vi "6_1.vi"() -> ()   [LabVIEW 2023, in "2025.lvlib"]
uses:
  2025.lvlib
  <userlib>/_OpenG.lib/string/string.llb/Trim Whitespace (String)__ogtk.vi
  <userlib>/_OpenG.lib/string/string.llb/openg_string.lvlib
panel:
  out "array w/ subset deleted":string[][](array[string])
  out "Numeric 2":i32
  out "Numeric":i32
  out "sum 2":u64
  out "Array 3":u64[](array[numeric])
  out "output 2":string
  out "number":u64
  out "error out":errorcluster
  out "output 1":string
  out "transposed array":string[][](array[string])
  out "Character Array":string[][](array[string])
  out "Array 2":string[](array[string])
  out "Array of Strings 2":string[][](array[string])
  out "sum":u64
  out "Array":u64[](array[numeric])
  out "Array of Strings":string[](array[string])
  in  "Boolean":bool
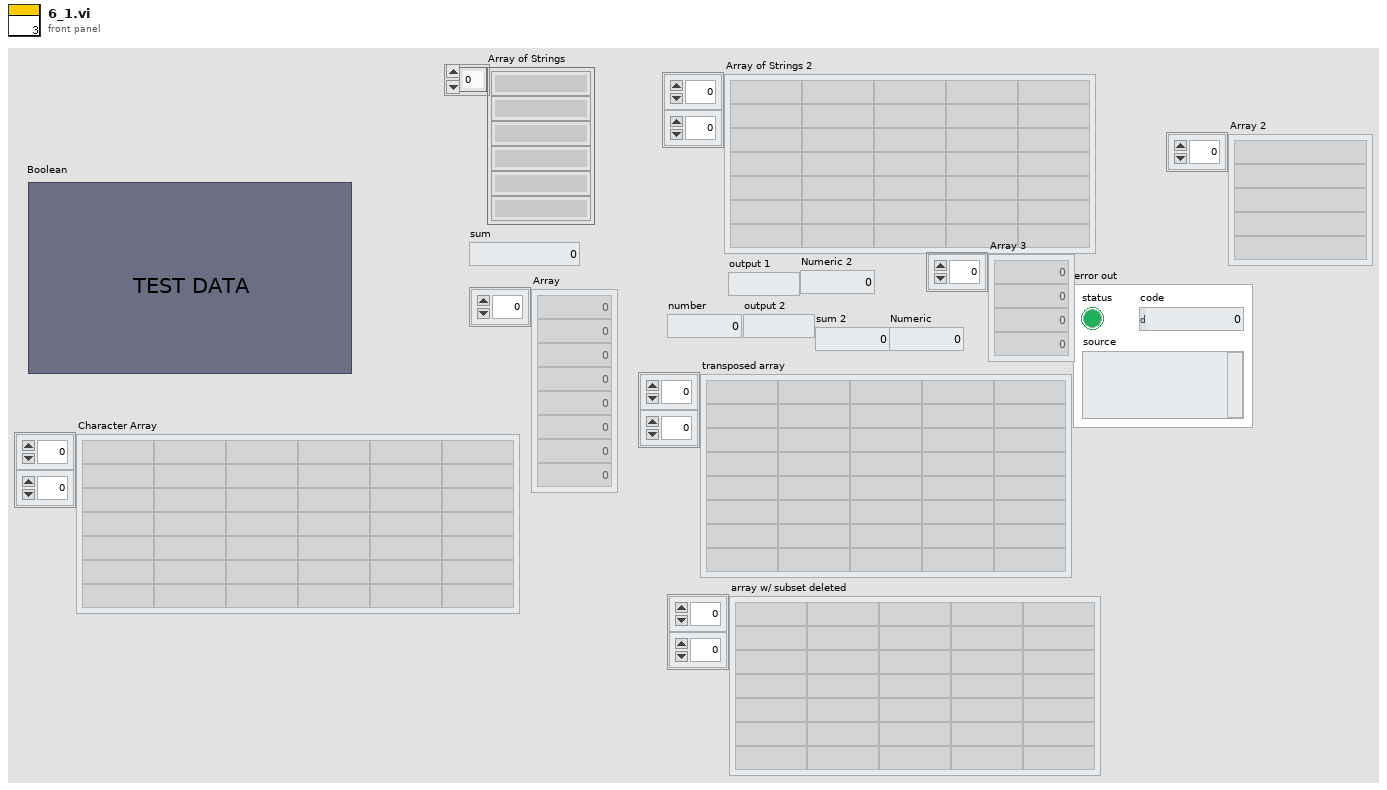
[diagram p1: front panel]
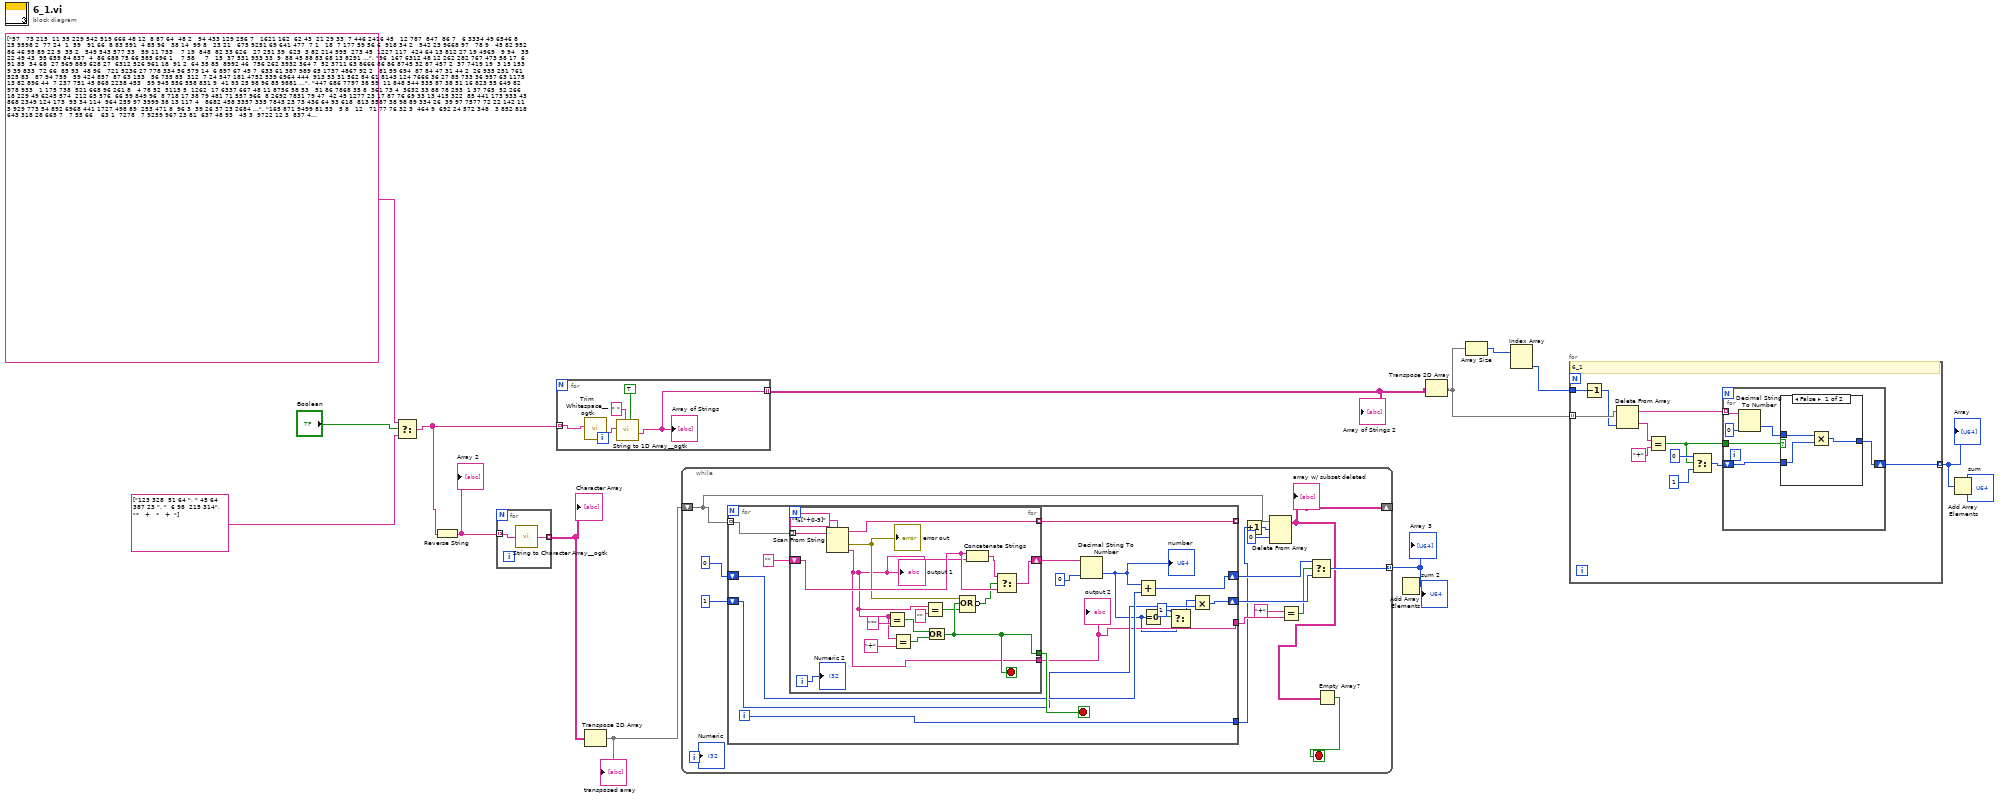
[diagram p0: block diagram]
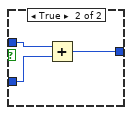
[diagram p2: hidden frame]
diagram:
  n1 = Select(t=string[] ["57   73 215  11 35 229 542 519 666 48 12  8 87 64  48 2   94 433 129 256 7   1621 162  62 43  21 29 33  7 446 2416 45   12 787  847  86 7   6 3334 49 6546 8  25 9598 2  77 24  1  59   91 66  8 83 591  4 85 96   38 14  99 8   23 21   675 9251 69 641 477  7 1   18  7 177 59 56 6  918 34 2   942 23 9668 97   78 9   45 82 952  86 46 95 89 22 9  35 2   549 543 577 33   59 11 733    7 19  848  82 33 626   27 251 39  623  3 82 214 595  273 45  1227 117  424 64 13 812 27 19 4969   9 94   35 22 49 43  95 659 84 837  4  86 688 75 66 585 696 1    7 58     7   15  37 531 933 33  9  88 45 88 83 68 13 8291 326 14  69   4 5   613 874 245  76 799 183 42  257 391  2  56 95 43 15    5  4 24  966  3 412 5  264  52 15 3  434 242  191 82    9   1 515 846   922 76   15 6281   1 59 73  9    62 18  74 82 72 6  844  8  18  898   7   33 847 4977 38 24 23 39  7 5561    9 9  93   9 417 971 77  26 89  7 5641 1  211 7  459 47 9   6    32  8 975 58 29 143 372 955   1 968  9 452  5 5  71  42 29 172 54 77  76   469  1 4352 956 3669 926 8381  1  916   2 44 536 161 3    78  4 4546 8   53 866   74  86  4 2  478 32 8   917  533 75 869 9   33  93 583 67 434  66 926  12 737 981 4    8 536  2674 3    6332 1515   4 24  1 982 717 41 26 64 5  53 432 662  815 486 147 6   4 87 84 2712 4   793  89 2164 539 675   59 96 6888  1 373   1  16 721 97  54 16 759 66 8  5    948 17  6  8  45 923 4664 36  4 62 624 73 494 73 171 312 98  3 288 63    9 7351 69    44  4   8   3  2 414 942  62  1  3 528 83 779 158 1  781 27  946 879  21   8 895  24  327 49 39  33 2361 58 15 325 89 82 76   99 845 7981 241   6 3377 12 72 543 837 5647 566 298 6293    3 8974 456 957 2    871 2197 993 13   66 8853 6  1  246 5    9   97 56 552  233   8 955 86 52   3 9   4  5  57 62 239 3  57 339 7  754 43 55 8663 242  68 33 79 4617  3 9  782 37 119 1  24  865 319 5   16 335 824   5 591 14   1   1 483 39   7 478 99 3815 97  77 176  5 2499 4935  52 841  71 181 96  4 76 59 888 61 3363 21 565  7 7   38  591 79  4    1 16   37  27 58 79  77 1   578  75 54 6   55  7 142  41   19 97 753 918 786 94  2     4  3 882   6 4352 92 975  7 691  268 74 819   54 6   2  54   94 6341 35  738  73 89 6  53 19  6791 63 339 12 78 2   9 35  697  56 132 84 95 8611 37 16 144 8  66 61 512 2  919  613   1  9 95 68 489 225 576 222 9  769 3374 95 35 53 25 222 638 4    1 84 1  56   8 57 182 443 797 136 9    9   8 53   53 3  3721 79 15 583   16 335 23 7158 564  4  9 65 72 3719 891 683 3769  83 233  771 51 811 65 4  7567 5842  93  83 23 32 935 77   6976 26  52 53 549 8936 76 1  6   5  6   872  7 83 3376 512 61 59 354  5367  4 9434 56 67    5 9  32    3 5846  7 5  9    98 535 12  37   1 7846 62 41 73 63 894 3   9 635 3724  96  16 11 51 69 495 15 97 54 536    5 987 82 353  6 939 72 389  53 52 11   4 344 3   782 5    228 657 328 543  516  4 348 5629   13 447 666   8 95 832 291 411  74  19 39 483  9 88 11   46 37 56  74 25  6683 1157 616 73 9  86  71 71   59 7    4  37 14 348 559 76 987  78 55 5  14 443 7682 1   1721 516 91   836 464 634 44 7428 64  471 218 646   9  2 57 9    183 71 46  17 917 12 13   235  5 488 4566 953 191 42  1 481 63 9  344 28  253 116 19  74 12 57  8 1697 15 9414 54   25 213 33 515 95 11  6183 23 814  396 4  66 663  7 29 266  81 335 84  5 5284 7  23 63 454 778 3926 696 4    74 84 2584  95 763 528 565 7  962  2  12 64 71   9 5  13 272 374 73 17 58 985 2   14 47 56 5    27  69   23 48 24  229 75 8429 7546 98   6 86 9974 151 6918 77 798 12 862 565 7157  92 848 45  79 48 69 741 96  45   818 35 96 9246 542 9486    9 152 9  41 881  38 292  77 6   3  9  4  5  81 94   62 327 97  35  3824 426 3   7    88 537 543 921   6 95  471 113   36 3  31 761   7 7934 8787 317  2 7996 35 38 649 24  29 6717 53 25   892 24 846 74  4 661 54 2238 6993 61 93 16   6 962 78 67 4   958  45 395 393 2   95  338 38   865  7 7318", "96  167 6312 48 12 262 282 767 473 58 17  6 91 85  34 68  27 569 889 628 27  6312 526 961 18  91 2  64 35 85  8992 46  756 262 3932 364 7  52 3711 63 8666 86 86 8745 32 87 457 2  37 7419 19  3 15 153  9 39 833  72 66  85 93  48 96   721 5236 27 778 334 56 579 14  6 897 67 45 7  633 61 387 989 65 1737 4867 92 2   81 59 694  87 84 47 31 44 2  26 935 251 761 525 83   87 94 759   59 424 857  87 63 153   56 735 85  312  7 24 547 181 4752 539 6964 444  913 53 31 562 84 61 8143 124 7666 36 27 85 733 36 957 63 1175 13 82 896 44  7 237 751 45 868 2238 453   59 945 556 558 831 9  41 93 25 98 96 85 9881 836 761 55  79 85 3122 327 2117 83 386 292 88  457 235 72  99 94 99 45  266 44 85   55 68 72  8  587 848 7  8   16 811 2697 362  48  66 413 7369  584 21  796 7819  41 57 31  93   39 52  26 57 82 89 657  1  217 243  99  817 648 5217 41 63 14 61 38 6165 4754 7  98 783 626 153 24 478 39  6 6187 56 361 47 468 49 37  38  495  1 873 26 65  36 641 479  51 472 96 192  9 1  39  18 24 211 49 72  31  3878  8 3547 33  5588 964 1169  6 7481  28 75 682 321 4    59 28 1821 87  92 154   74  91  9 59 92  27 93  419  292 31 553 99  76  62 733 54 765  23 669  44 478 84  8   56 679  7426 98   9569 7284 678 55  6 785 114 5  66 34 3  74 527 118  151 146 547 81 34 23 93 9478 1   965 824 9313 768 59   974 38 3868 82 571   9  55 249 664 74 28  29 37 23 364  888 71  2 76 756 648 8179 59  9 41 781 44 838 33 132 492 37 23 577 9197  2 3447 3261 626  2 849 759 51 993 254  77 37  8 716 79 198 419 42 242 27 1356 2515 15   4 162  18  675 47 96  46 581  43 91 393 25 93 87   26 483 4614 337  45   99  7 84  63 888 7676 236  95 5241    6 5181 142 914 5952 634 4579 685 57 7715 3659 4  8  662 97   1 1942 47 6876 249 347 491 95 79   7 8   18 3  62 52 537 51 65 532 17  81 97 81 1324 611  24 32 49 7996  3 92 516 19 472 8  31 6255  15 4   18 773 285 794 317 21   9   5 252 51   5 41  53 2396 53 489 764 88 3767  919  85 518 842 633 92  3 19 58 246 97 9315 33 523  7 611 89   31 755 77  65 6659 38 946 17 68 513 23  478  62 35 843 54 85 464  87 3387 25  99 298 497 113 126  44 55 71   27 7164 59 525  2 416  327 24 285 7122 62  2  636  53 4842 12  365  28 43 6  53 32  489  24 828 77 22 12  9 812 793  31 221 81 79  832 97 94 834 7  52 96 976 15 9616 899  77 49 14 35 839 921 398 926 5  474  615 53 77 94  8  83 736 43   8 43 1  63  63 19 382 882 316 222 41   34 36 74   95 9  2138 15 36 818  281 536 95 7653 631 22 97 39 11 4482 784 978 6338  47 2737 235 31 495 88 4   814 5282 355 414 41 73 942 158  7598 32  19 55 323 398  92 95 98  33 59  619  7 56 6231 926 68 28 284  6973  6 5937 11 194  72 3  652 319  577 72 25 216 689 658 27 828 476 9578 67 94 65 35 442 12 72 843 5432  61  16 94 98 46 382 56 34 31 754  126 928 42 522  9 439 77 849 826 81 22   4 422 76  478 629  563 315 856  41 4157  1 86  1146  381  33 669  78 91 117 324 587 753 495 57 591  5 66 449  66 82 94  29 592 4254 7359 413 67 6  72  25 587  61 5    3 358 36 177 478 34 318 374 12 7  21 288 7239 459 5779 678 967  995  12 994 44 3931 69  933 635 439  88 88 32 5    986 53 171 45 454 58 8849 199  9 942 1211 724 793 21 76 932 67 75 291 75  835 292 92  59 55 31 84 1749 72 2246 74   58  99 29 225 49 882 4972 98 425  251 33 61 932  2 14 543  62 325 21 19 2335 8  47 16 324 194  786 966 63  117 64 4588 617 415 763 977 98 185 84 926 28 14  11 6  18 252 529 2  96 43 136 37  53 93 13 725  39  11  167 98 49  718 71  246 1646 45  44 77 9887 577 9281 67 894 16 514 122 2352 453 662 95 426 99 16 919 323 797  353 17 63 2163 595  644  564 758 26 73 566 333 523 143 571 5  27 53 5  85 848 285 526 545 149 9986  38 71  6167 6  784 619 527  77 39  659 1373 238 3  15 163  23 5592 6824  92  5 3299 62 71 721 469 39 1284 62 53  6314 68 51  84 56 876 23 6488 3433 55 12 85  45 353 64 96 52  567  62 811 948 46  61  94  1276 456  1  979", "447 686 7797 38 59  11 848 544 535 87 38 51 16 823 55 649 82 978 933   1 175 738  521 668 96 261 8   4 78 52  5115 5  1262  17 6337 667 48 11 8756 58 53   51 86 7868 35 8  361 73 4  3632 33 88 78 293  1 37 765  52 266 18 229 49 6245 574  212 65 576  66 59 849 96  8 718 17 38 79 481 71 557 966  8 2692 7831 79 47  42 45 1277 23 17 87 76 69 33 13 415 322  85 441 173 933 43 868 2349 124 173  93 34 114  964 259 97 3999 38 13 117 4   8682 458 3357 335 7843 23 73 436 64 93 618  813 5587 38 98 89 334 26  39 97 7577 72 22 142 11  5 929 773 54 892 6968 441 1727 498 89  253 471 8  96 3  39 26 37 23 2684 779 333 13 667 83 3443 247 7239  1 942  73  8  398 39  72 267 72 14 629 656 92 52   94 37 7   4   61 851 3  55  67 852 8193 3439 37  38  53 3651 2548 22 5211 4494 226 96 549 6396  4 2   14 51 36 59 229  33 423 236 116 7857 288 473  75 71 49 26 42 13   3883 99 71 278 689 29  98 712 83  7  766 59 949 72 566 59 888 183 397  2 692 1   2  68 188 551 794 29  97 791 61 69 941 79 15  41 49 997 894 6199 52 4449 9   3257 142 1448 29 9852 971 34 866 684 721 854 63  679 22  22 712 3935  35 37 53 86  62 785 116 9146 64 926 974 31  73 845 36 4585 55  26 742 332 46  5  782 6599 1591 2648   11 413  443 75 62 686 614 2  73 67 4  28 227 883  132  18 166 68 57 65 16 87   64  373 895 1781 523 95  4957 66 6562 23 953  67 682 541 547 64 89  16 1  47 358 2155 51 42 99 483 579 3433 42  1 27 385 45 561 83  94 624 49 37 235 3411 35 9558 6167 447 16 591 221 85 445 387 251 52 64 866  6 623  29 33 12  59 4563 4941 525 37 4873 236 593 83 633 32 547  13 64 468 34 96 51  298 228 3375 316  38   35  2 72  78 363 9946 613  33 2983 9714 5791 66  447 4778  84 3384 81  29 5613 224  48 65 17  169 12 1291 19 3643  89 143 154 19 35   2 995 96 9  44 7  696 39 18 315 94  98 47 83  354 1636 73 33  4 36   73 14   7 16 537 33 81 7379  55 286 28 282 98  352 997 776 82 884 882 35 829 47  83 7133 62 969 543 22 5772  379 616 28  696 464 89  7 72 88 697 1  9869 68 213 91 196 622  24 166 45  38 7614 27 363 91 67 989 383 121 248 48 288 92 58 626 322 1196 32  32 971 524 956 751  65 18 54   11  442  2 21   2 994 1381  4 469 8368 692 48 954 469 5349 191   2  51  7 56 99 987 56   87 47  66 53 49  9 141 584 169 947 95 85  563 51 74 297 88 34 26   6 28 7254 847  41 56 84 56 424 314 97  323 43 326   73 95 17 69  8  54  76 941  4 54 84 23  61 49 996 917 97  857 8743 49 21 5884 45 84 3937  7 94 581 5435 246  4 4291 657 95 97  7 9   118 147 584 8217 718 5333  22 21 811 69 47  634 7366 676 888 69 14 939 541  6454  4 941 29 614 68   37 32 859 59 265  53 38 54 6997 939 33 56 794  881  44 4162 26 725 258 47 694 368  753 28 93 423 212 42  73 782 372 3676 17 62 79 64 834 76 49  49 523  227 835 84 53 65 447 42 3  84 78  6777 137 57   7  6 386 72 818 959 56 15  61 532 213 369 1133 475 824   5   5 8751 91 78  5171  872  81 4277 91 2  963 676  72 426 632 36 381  6 44 9124  3 88 23 414 556 5136 83   543 72 2  61  82 9261 54 985  4 512 25 73    5 1    1 579 47 49 45 811  976 975 2823 363 7985 458  64 571 81 2663 942  52 56   76 668 25 85 973  566 41 467 93 834 83 5426 681 85 174  316 573 93  49 12 532 55 99 865 542 281 29  866 85 29 81 12 3665 77 1994 659  86  35 26 57  54 767 3531 27 44  7773 32 68 914 57 2  127 127 843 55 48 9358 83 47 95 865 327  266 515 73 2296 99 4218 319 26  286 69  34 652 71 719 32 78 867 99 3  967 147 1  65 39 928 588 36 23  3 773  868 49 1981 62 36  436 16   68 2413 37 623 18  286 263 9775 1   59 62 298 278   51 297 228  8 738 88 97 844 544 8699 5   35  2 8257 359  123 6839  95 15 21 368 335 587 353 461 65 46 24 65 24 619 137 653 858 134  877  76 735 3314 3  148  23 87   45 756 432 2451 672 1  35 173  97 2575  361  24  4 2913 67 94  61 974 29  685 17 961 1214 61 29  26 83 378 98 184  8211 9  11 462 74 573 86 77 178 564 928  42 197 486 536 95  3348 171 49  459", "165 871 9499 81 53   5 8   12   71 77 76 32 3  464 9  692 24 572 348   3 852 818  643 318 28 665 7   7 55 66    63 1  7278   7 9259 967 23 81  637 48 93   45 3  9722 12 3  837 43 2  1494 57 58 25 177 97 54 2917 4  475 41 564 95 4118 715    9 13 618  45 44 146 43 55 7   18 66 48 7   6  754  73  1 9852 9934 84 385 34 89 5512 4  23 34 86 58 86  7 117 284  45   5 876 721 45 48  2444 881 25  635 69 34  6146 96  95 9592 26 55 384 5   6749 695 3749 714 8851 49  7 232 33  2 78   214 3388 71 15 33 763 66   6 99 4948 31  7 958 99  2 29  497 84 199 9575 894 2924 795 17  532 548 85 7  7  12 24 63 4  6626 71  725 48 282 99 8363 526 9521  4 64    9  6 3362 74  21 643 1  74 387 697 58 761   8 76 8   17   5 323 6  46   3 757 1245 9261 31 716   9 2737 2546 6  6697 9661 682 36 454 9846  8 3  681 67 27 29 2139 38 517 939 735 1532 374 599  17 31 31 94 92 86   6785 86  9 836 853 68   5 814 12 49  541 32 11  58 43  38 544 788 738 29 8   2   3   6 245 5   754 77  72 184 38 62 771 84 43  16 16 419 553 4382 65  732 7     91 653 63   66 5328 178 37 557 7   868 399 67   86 166 25 744 8795 585 62 32 95   4 341 376 3583 96 628 994 639 97  61 84 3816 47  91 395 784 53  84 886 9945 225  4277   27 5    365 5  81 528 69  3  85 77 24 22 884 2321 449   2 188 38 56 38 29 8    424 95  329 852  152 92  5857 52  653 88  53 532 357 237 813  8 22  31 8  91 341 9294 24 67 49 819 816   96  2 69 45 3   85 445 9   95 947 49 99   7 6329 11  795 9143 613 12 767 787 51 22  388 258 76 85 122  3 966   6 55 37  58 6764 8243 353 51 4153 481 499 28 398 6  82   14  4 46  99 24 32 3192   5 83   86  796   71  5 65  54  13 9683  36  48 8159 7158 53   21  235 1899  85  918 71  78 1617 982  16 33 5   968 35 7641 59 9415  85 686 9   29  8 257 199 66 34 88 4  726 49 74 115 63  41 14 83  988 6184 97 61  1 6    42 93   5 4    3 28 3  1798  46 691 27 6   87  832 711 434 12 354 815 53 676 21  8  7454 69 199 321 75  263   23 878 15  816 999 6  18 54 84 697 5  66   59 535 67 782 431  28 674 28 148 5267 28 816 33 54 686 497 819 667 34 345 9  71 336 695 1984 54  74 13  291 151 258 912 89 54  481   58  9 4   23 611 3335  8  27 1692 412 11 651 385  486 793   9 955  2 43 26 529 75   47 81  52 41 11 19 962 75  176 758 9  19    5 33 77 33  86 97 53   6 37 2491 636 852 73  9 19 867  75 79   49 53 485   14 47 89 6   9  82  56 621 21  6 65 68 767 43 76  728 25  41  2753 86 54 3553 6  85 7644  2 15 351 7374 82   3 5364 566 11 59  4 3     4 526 485 8554 494 9664   8 33 49  79 67   32 683  724 149 42 3  628 9998 2     4 523 68 325 19   96 64 714 73 754  88 83 7  4418  16 32 61 2726 28   46    7 73 364 424 25 277 245    8 28 36 113 493 66  2  916 863 6118  6 35 19 87 54  36 73  85 37   852 925 41  5 31 325 8  1  87 2   2323 898 16   7 35 656 18 688 319 13 28 469 825 334   2 9842 965 916   5   7 4724 31 18  193  8873  81 7662 33 3  217 372   4 986 951 1  41  86 36 9548  1 56 99 141 336 4757 35   175 71 72 45 851 8436 64 239 87 694 46 3     9 3    6 895 51 96 4   88    1 673 687  185 5277 587   9 6   23   56 458   1 23    4 827 63  2 7774 144 38 254 14 289 47 1542 497 38 19   948 511 7   66 17  88 5  46 498 168 658 17  169 99 56 1  55   56 79  651 1666 91   1 64 5   57 737 452  21 1   6919 21 54 931 85 3   14 738 354 45 79 2333 12 62 17  81 347  381  42 24 6465 28 2524 375 9   263 6   78 26  44 454 5  43 817 85 3  28  129 9  49 83  73 382 27 76  4 1321 891 43 8578 35 363 4   38    3  172  4 685 98   49 6   4594 3   34 72 878 435   12 967 51   1 984 93 1  8   421 7776 2    2  4  386  52  784 4968   9 75 6  569 611 722 936 345 82 55 15 22 13 986 179 633 837 443   72   5 416 1249 5  146   1 2   196 835 596 8915 992 99  4  49 587    1    3   4 73   33 84 23  82 938 97   67  9 489 1725 6  86  97 92 467 44 88      7 6  88 955 73  85 2  32 389 548 987  74  53 375 189 46  2373   5 99  818", "+   *   +    *  *  +   *   *   +   +  *  *  *  +   *  +   +  *   +   +   *   +    +   +   +  *   *  *  *  *   +    *  +    +   +    *   *  *  +    +  +    *  *  +    *  +  *   *  *  +    +  *  *  *   *  *  +    *  +   +  *   +  +    +   +    +  +   *   *  +   *  *  +   *  +  *  *   *  +   +   +  +    +    *  +   *  +  +    *  *  +  *  *  +  *  +   *   *   *   +   +   *  *   +    +   *   *   +  *   +    *   *  +    +  +  *   +   +    +   +    +   +    *  *  +   *  *  +    *   +    *  *  +  +   *  *   *  +    *  +  +   *  *  *   *   +  +   +    *   +    *   *   *   *   +  *  *  +  *  +  *  +    *   +   +  *   *  +    +   +    +  +   *   *  +    +   *  *   *  *  *   +   *  *   +   *  +   +  +   +   *  *  *   +   +    +    *  *   +   +    +    *  +    +    *   +  *   +    *  *  *   *  +  *  +    *  *   *   *   +    +   +    *  *  +  *  *  +    +    +  *  *   +   *   *  *   *  *  +    *  *   *  +   *  *   *   +   *  *   *  +  +   *   *   +   *   *  *   *  +  *   *  *  +   +  +   +   +    *  +    +   +    +   +    *  +    +   *  +   +   +   *   +  +    *   *  *   +    +   +  *  *   +  *   *   +    +  +   *   *   +  *   +  +    *  *   *   *   +   *  *   +    +    +    +    +    *   *  *  +   +   *  *  *  +  *  +   +    *   *   *   +  +  *  +  +    +   +   *   +    +   *   +    +  +    *  +   +   +   +   *   *  +  *   *  +  *   +    *  +  *  +   *   +    *  *  +  *   +  *   +  +   *   +  *  *   +    +  +    +    *   +  +   +   *  *   *   *   *  +  *   *  *   *   *  +   *  +    +    *   +  +    *   *   +  *   +  +    *  *  *   +  *  *  +    +   +    *   *   +    *  *  +   +   +    +   +   +    +    +    *   +   +    *   +    *   +  +    +    +  +  *   *   *  +    *  +    *   *   +   *  +  *   *   *  *  *  *  *   *  *  +   *  *   +  *  +    +    +  *  *  +    +  +  +   *  +   +  +  +    *   *   *  *   *   *   *   *   +  *   *   +  *   +   *  +    +  *   *   *  +    +    *   +   *   *   *  +  *  +  *   *  +    +  *   *  +   *   +   *   +  +   +    *  *   +  *  +   *   +   *   +  +   +  +  +   +   +    *  *   *   *   +   *   *   +  *   *   +    *  +   +  *   +    *  +   +    *   +  *   *   +    *   +   +   +  *  +  *   +    +  +   *  *  *  *  *   *   +   *   *  +  +    *  *  *   +  +  *  *   +  +    *   +   *  +  +  *   *   *   +   *  *   +    *  *  +  *  *   *   +   +  *  *  +  *   +  *   *   *   *   +    *  *  +    *  *  +    *  *  *   +    +   *  +    *   *  +  *  +  +    *   +   +    +   +    *   *  +   +  *  +    +    *   *   +  *  *   +    +    *  *   +  *   +    +  +  +   *  +   +   *  +  +    *   *  *  +    +    *  +    *  +   *   +  *   *   +    *  *  +   *   +   *  *   *   +    +  *  +  *  *   +  *  +   +    *   *   +  +  *  *   +  +  *  *   +    +   *  *   *  +   +  *   *   +  +  +   *   *   *   +    *   +   *   *   +    *  +   +    +    *   +    *  +  +   +   *   +   +   *  *   +  +  +    +  *  +  *   *   +    +    +   *  +  *  +   +    +  *   *  *   *  +   +   *  *   *   +  +  +  *   +    *   +    +   +    *   *   *   *  +    *   +   *   *   +   *  +  +    +   +  *   *  *   +  +    +   *  +   +    *   *   *  +  *   +  *  *   *   *   +   *   *  *  +  *  +    +  +    +    *  *   *  *   +  *   +    *  +   +    *  *  *   +  +  *   *   *   *  *  +    +  +  *  *   +   +    +   *  +    *  +    *   +   *   +   *  +   *  +   *  *  +   *  +  +   +   *  *  +  +   *   +  +  +  +    +   *  +    *  *   *   *  +    +    *  *   +  +    *   +    *  +   *  *   *   +    *   *   *  *   +  *  +   *   +    *   *  *  +    *   +    +    +   +  +  *   *   *   *   *   *  +  +  +  *  +   *   *   *   *   +    *   +   +    *  +   +   *   *   +   *   +    *   *  *  +   +   +    +    +   +  +    *  *  +   *   +  +    +  *   +    *  *   *  *  +   *  +    +    *  *  *   +  *   +  *  *   *   +   *   +   +   *   *   +    *   *  +   "], s="Boolean", f=string[] ["123 328  51 64 ", " 45 64  387 23 ", "  6 98  215 314", "*   +   *   +  "]) -> (s? t:f=w6:string[])
  n2 = Reverse String(1:w6) -> (0:w5:string[])
  "Array 2" <- w5
  n3 = for {
    tunnel: w5 -> [w17] mode=indexing
    tunnel: [w16] -> w4 mode=indexing
    n4 = call <userlib>:"String to Character Array__ogtk.vi"("Input String"=w17) -> ("Character Array"=w16:string[])
  }
  "Character Array" <- w4
  n5 = for {
    tunnel: w6 -> [w20] mode=indexing
    tunnel: [w18] -> w7 mode=indexing
    n6 = call-poly <userlib>:"Trim Whitespace__ogtk.vi"("String in"=w20) -> ("String out"=w19:string)  [unwired: 6 in]
    n7 = call <userlib>:"String to 1D Array__ogtk.vi"("ignore duplicate delimiters? (F=No)"=TRUE, "delimiter (Tab)"=" ", "string"=w19) -> ("Array of Strings"=w18:string[])  [unwired: 8 in]
    "Array of Strings" <- w18
  }
  "Array of Strings 2" <- w7
  n8 = Transpose 2D Array(2D array=w4) -> (transposed array=w3:string[][])
  "transposed array" <- w3
  n9 = while {
    shift-right: [w24] -> _
    shift-left: w3 -> [w26]
    tunnel: [w30] -> w2 mode=indexing
    i -> [w27]
    stop <- w23 stop-if-true
    n10 = for {
      tunnel: w26 -> [w51] mode=indexing
      tunnel: [w53] -> _ mode=indexing
      shift-right: [w46] -> w33
      shift-left: u64 0 -> [w47]
      shift-right: [w44] -> w32
      shift-left: u64 1 -> [w45]
      tunnel: [w43] -> w35
      tunnel: [w42] -> w28
      i -> [w42]
      stop <- w52 stop-if-true
      n11 = for {
        tunnel: w51 -> [w70] mode=indexing
        tunnel: [w69] -> w53 mode=indexing
        tunnel: [w56] -> w43
        tunnel: [w59] -> w52
        shift-right: [w62] -> w49
        shift-left: "" ("output 1") -> [w61]
        i -> [w57]
        stop <- w59 stop-if-true
        n12 = Scan From String(format string="%[*+0-9]", input string=w70) -> (remaining string=w69:string, error out=w60:errorcluster, output 1=w56:string)  [unwired: 3 in, 1 out]
        "output 1" <- w56
        "error out" <- w60
        n13 = Equal?(x=w56, y="*") -> (x = y?=w66:bool)
        n14 = Equal?(x=w56, y="+") -> (x = y?=w64:bool)
        n15 = Equal?(x=w56, y="") -> (x = y?=w54:bool)
        n16 = Or(x=w66, y=w64) -> (x .or. y?=w59:bool)
        n17 = Compound Arithmetic op=OR(w60, w59, w54) -> (invert w58:bool)
        n18 = Concatenate Strings(w61, w56) -> (w63:string)
        n19 = Select(t=w63, s=w58, f=w61) -> (s? t:f=w62:string)
        "Numeric 2" <- w57
      }
      "output 2" <- w43
      n20 = Decimal String To Number(string=w49, default (0L)=u64 0) -> (number=w40:u64)  [unwired: 1 in, 1 out]
      "number" <- w40
      n21 = Add(x=w40, y=w47) -> (x+y=w46:u64)
      n22 = Equal To 0?(x=w40) -> (x = 0?=w41:bool)
      n23 = Select(t=u64 1, s=w41, f=w40) -> (s? t:f=w38:u64)
      n24 = Multiply(x=w38, y=w45) -> (x*y=w44:u64)
    }
    n25 = Increment(x=w28) -> (x+1=w25:i32)
    n26 = Delete From Array(array=w26, length=w25, index (row)=0) -> (array with subset deleted=w24:string[][])  [unwired: 1 in, 1 out]
    "array w/ subset deleted" <- w24
    n27 = Equal?(x="+" ("y"), y=w35) -> (x = y?=w31:bool)
    n28 = Select(t=w33, s=w31, f=w32) -> (s? t:f=w30:u64)
    n29 = Empty Array?(array=w24) -> (empty?=w23:bool)
    "Numeric" <- w27
  }
  "Array 3" <- w2
  n30 = Add Array Elements(numeric array=w2) -> (sum=→"sum 2":u64)
  n31 = Transpose 2D Array(2D array=w7) -> (transposed array=w10:string[][])
  n32 = Array Size(array=w10) -> (size(s)=w9:i32[])
  n33 = Index Array(array=w9) -> (element #2=w8:i32)  [unwired: 2 in, 1 out]
  n34 = for {
    tunnel: w10 -> [w81] mode=indexing
    tunnel: [w72] -> w12 mode=indexing
    tunnel: w8 -> [w71]
    # "6_1"
    n35 = Decrement(x=w71) -> (x-1=w80:i32)
    n36 = Delete From Array(array=w81, index=w80) -> (deleted portion=w78:string, array with subset deleted=w79:string[])  [unwired: 1 in]
    n37 = Equal?(x=w78, y="+") -> (x = y?=w74:bool)
    n38 = Select(t=u64 0, s=w74, f=u64 1) -> (s? t:f=w73:u64)
    n39 = for {
      tunnel: w79 -> [w87] mode=indexing
      tunnel: w74 -> [w85]
      shift-right: [w82] -> w72
      shift-left: w73 -> [w83]
      n40 = Decimal String To Number(string=w87, default (0L)=u64 0) -> (number=w84:u64)  [unwired: 1 in, 1 out]
      n41 = case shown="False" w85 {
        tunnel: w84 -> [w90 w93]
        tunnel: w83 -> [w89 w92]
        tunnel: [w88 w91] -> w82
        frame False {
          n42 = Multiply(x=w90, y=w89) -> (x*y=w88:u64)
        }
        frame True {
          n43 = Add(x=w93, y=w92) -> (x+y=w91:u64)
        }
      }
    }
  }
  "Array" <- w12
  n44 = Add Array Elements(numeric array=w12) -> (sum=→"sum":u64)
